vi "GV frame counter.vi"() -> ()   [LabVIEW 2017]
panel:
  out "Framecounter":i16
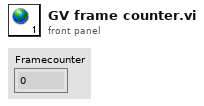
[diagram p1: front panel]
diagram:
